vi "mupCreate.vi"(8 "error in (no error)":errorcluster) -> (0 "error out":errorcluster, 3 "hParser out":u64)   [LabVIEW 2018, in "mupLib.lvlib"]
doc: "Opens a new muParser instance. Returns the muParser handle."
uses:
  mupLib.lvlib
  libmuparser-lv.dll
panel:
  # "Opens a new muParser instance. Returns the muParser handle."
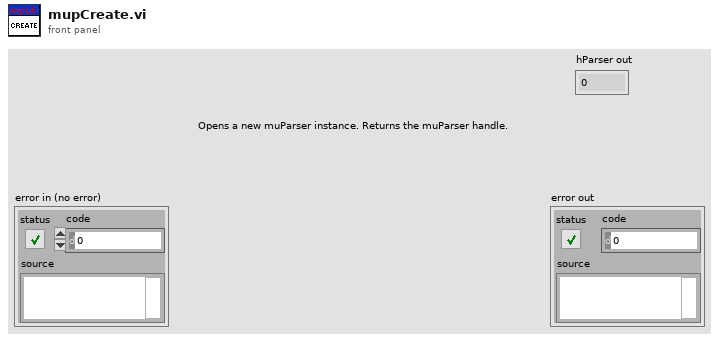
[diagram p1: front panel]
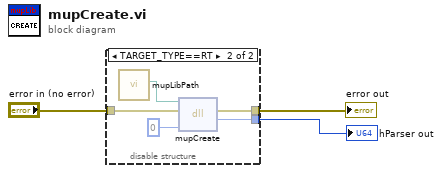
[diagram p0: block diagram]
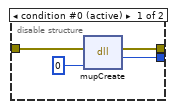
[diagram p2: hidden frame]
diagram:
  n1 = disable-structure shown="TARGET_TYPE==RT" {
    disable-tunnel: "error in (no error)" -> [w7 w12]
    disable-tunnel: [w6 w11] -> w2
    disable-tunnel: [w5 w10] -> w1
    frame condition #0 (active) {
      n2 = dll-call lib="C:/Users/leonidas/Documents/GitHub/LV-muParser/mupLib/libmuparser-lv.dll" fn="mupCreate"(error in=w7, "nBaseType"=0) -> (error out=w6:errorcluster, "hParser"=w5:u64)  [unwired: 3 in, 1 out]
    }
    frame condition #1 {
      n3 = call "mupLibPath.vi"() -> ("libmuparser path"=w8:path)  [unwired: 11 in]
      n4 = dll-call lib="C:/Users/leonidas/Documents/GitHub/LV-muParser/mupLib/libmuparser-lv.dll" fn="mupCreate"(path in=w8, error in=w12, "nBaseType"=0) -> (error out=w11:errorcluster, "hParser"=w10:u64)  [unwired: 2 in, 1 out]
    }
  }
  "error out" <- w2
  "hParser out" <- w1
